vi "Generate Simulated Data.vi"(6 "Acquisition":refnum<queue>, 8 "error in (no error)":errorcluster, 10 "Longueur d'onde":dbl) -> (0 "error out":errorcluster, 2 "Data Out":variant[](array[variant]), 3 "Disconnected":bool=TRUE)   [LabVIEW 2018, in "Acquisition.lvlib"]
doc: "Generates sample waveforms according to the signal type in the HW Config input."
uses:
  Acquisition.lvlib
  support/Message Queue/Message Cluster.ctl
  <vilib>/DAQmx/write.llb/DAQmx Write (Digital 1D Bool NChan 1Samp 1Line).vi
  <vilib>/DAQmx/read.llb/DAQmx Read (Analog 1D Wfm NChan NSamp).vi
  <vilib>/Analysis/baseanly.llb/Mean (DBL).vi
  <vilib>/Analysis/2dsp.llb/2D Convolution (DBL).vi
  <vilib>/DAQmx/create/channels.llb/DAQmx Create Channel (DO-Digital Output).vi
  <vilib>/DAQmx/miscellaneous.llb/DAQmx Fill In Error Info.vi
  <vilib>/DAQmx/create/channels.llb/DAQmx Create Channel (AI-Voltage-Basic).vi
  <vilib>/DAQmx/configure/timing.llb/DAQmx Timing (Sample Clock).vi
  support/Message Queue/Enqueue Message (Single).vi
  GlobalVariable/GlobalPowerByTime.vi
  GlobalVariable/GlobalSet0.vi
  GlobalVariable/GlobalPosYbyTime.vi
  GlobalVariable/GlobalPosXbyTime.vi
  GlobalVariable/GlobalProfileByTime.vi
  GlobalVariable/Globalt0.vi
  GlobalVariable/GlobalTensionByTime.vi
  GlobalVariable/GlobalTemperatureByTime.vi
  GlobalVariable/GlobalTimeStep.vi
  <vilib>/gmath/interp.llb/Create Mesh Grid (2D) (x,y arrays).vi
  <vilib>/Analysis/NI_AALBase.lvlib
  support/Message Queue/Message Queue.lvlib
  <vilib>/gmath/NI_Gmath.lvlib
  <vilib>/Analysis/NI_AALPro.lvlib
  <resource>/objmgr/daqmx.rc
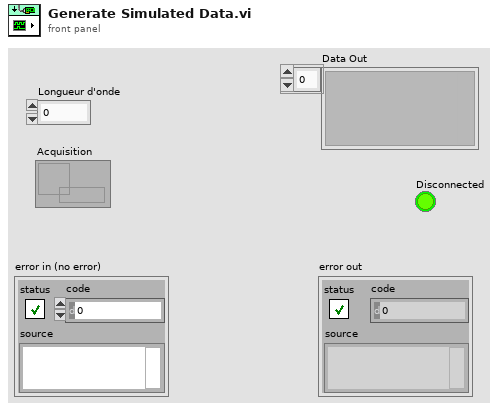
[diagram p1: front panel]
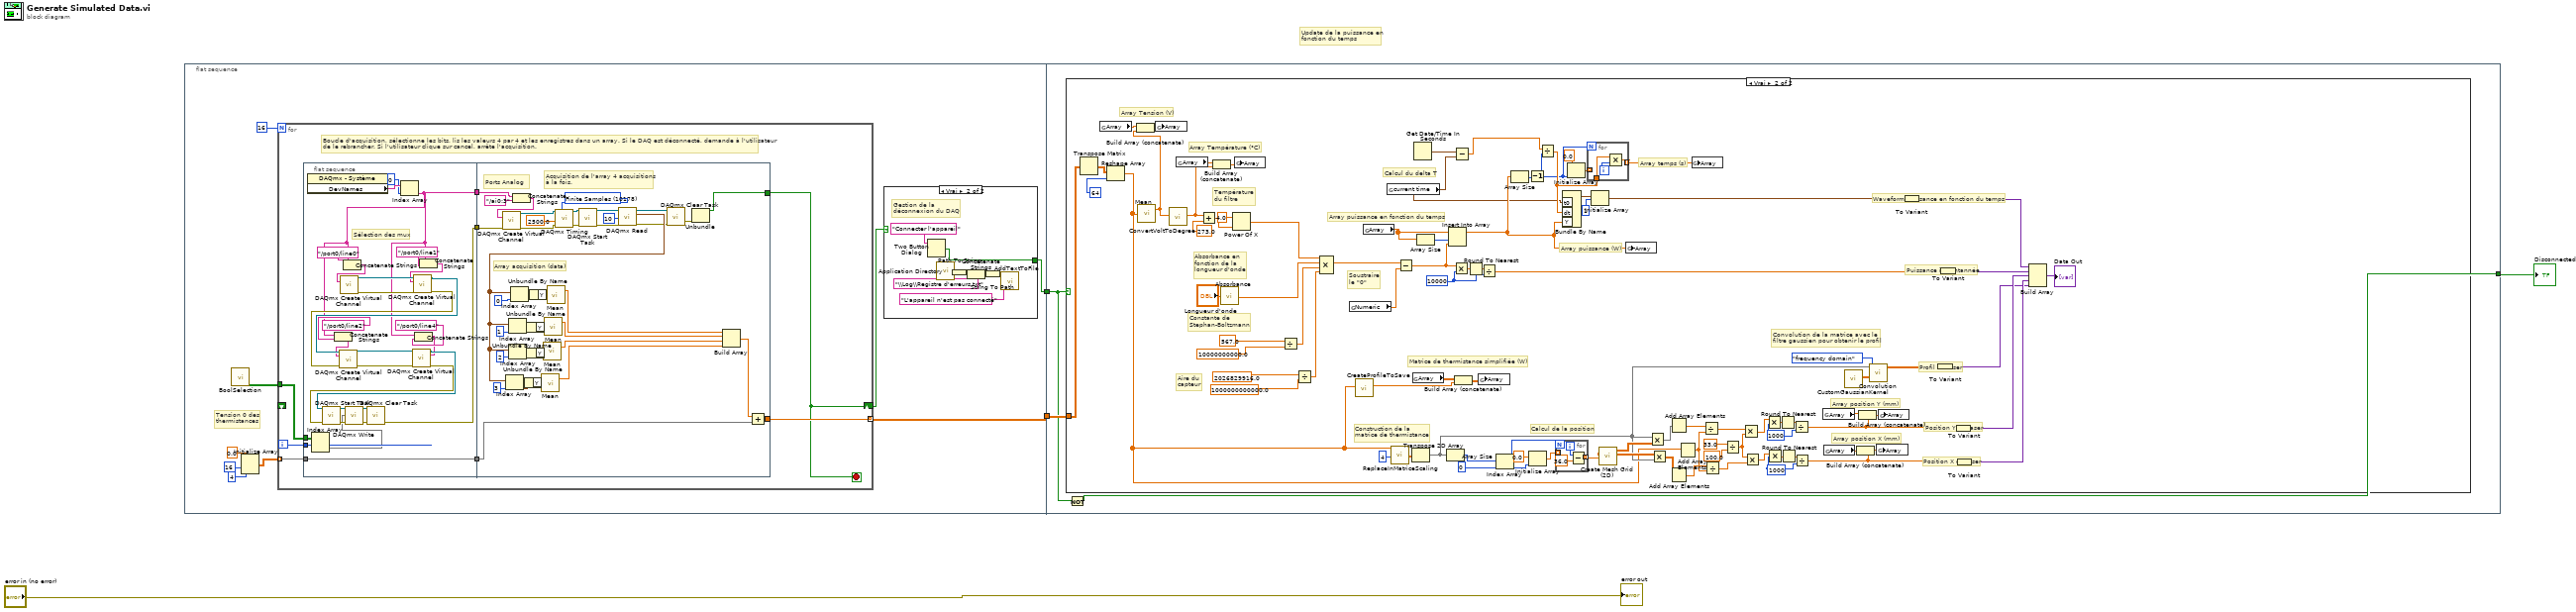
[diagram p0: block diagram]
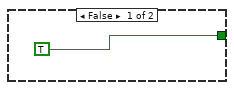
[diagram p2: hidden frame]
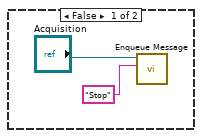
[diagram p3: hidden frame]
diagram:
  # "Update de la puissance en\nfonction du temps"
  n1 = flat-sequence {
    tunnel: [w11] -> w3
    tunnel: [w10] -> w2
    tunnel: w3 -> [w98]
    tunnel: w2 -> [w97]
    tunnel: [w96] -> w1
    frame #0 {
      # "Tension 0 des \nthermistances"
      n2 = call "BoolSelection.vi"() -> ("BoolSelection"=w12:bool[][])  [unwired: 11 in]
      n3 = Initialize Array(0.0 ("element"), 16 ("dimension size"), 4 ("dimension size")) -> (w6:dbl[][])
      n4 = for {
        N: 16 -> [_]
        tunnel: w12 -> [w28]
        tunnel: w6 -> [w26] mode=indexing
        tunnel: [w25] -> w11 mode=indexing
        shift-right: [w24] -> w5
        shift-left: _ -> [_]
        i -> [w29]
        stop <- w24 stop-if-true
        # "Boucle d'acquisition, sélectionne les bits, lis les valeurs 4 par 4 et les enregistres dans un array. Si le DAQ est déconnecté, demande à l'utilisateur \nde le rebrancher. Si l'utilisateur clique sur cancel, arrête l'acquisition."
        n5 = flat-sequence {
          tunnel: w29 -> [w44]
          tunnel: [w55] -> w30
          tunnel: w28 -> [w43]
          tunnel: [w42] -> w27
          tunnel: w26 -> [w42]
          tunnel: [w31] -> w23
          tunnel: w30 -> [w87]
          tunnel: w27 -> [w66]
          tunnel: [w68] -> w25
          tunnel: [w69] -> w24
          tunnel: w23 -> [w63]
          frame #0 {
            # "Sélection des mux"
            n6 = property class="DAQmx - Système"() -> ("DevNames"=w41:tag[])  [unwired: 2 in, 2 out]
            n7 = Index Array(array=w43, index (row)=w44) -> (element=w56:bool[])  [unwired: 1 in]
            n8 = Index Array(array=w41, index=0) -> (element=w31:tag)
            n9 = Concatenate Strings(w31, "/port0/line2" ("string")) -> (w34:string)
            n10 = Concatenate Strings(w31, "/port0/line0" ("string")) -> (w39:string)
            n11 = call-poly <vilib>:"DAQmx Create Virtual Channel.vi"("lines"=w39) -> ("task out"=w51:refnum<k21>, "error out"=w52:errorcluster)  [unwired: 13 in]
            n12 = Concatenate Strings(w31, "/port0/line4" ("string")) -> (w32:string)
            n13 = Concatenate Strings(w31, "/port0/line1" ("string")) -> (w36:string)
            n14 = call-poly <vilib>:"DAQmx Create Virtual Channel.vi"("task in"=w51, "lines"=w36, "error in"=w52) -> ("task out"=w50:refnum<k21>, "error out"=w49:errorcluster)  [unwired: 11 in]
            n15 = call-poly <vilib>:"DAQmx Create Virtual Channel.vi"("task in"=w50, "lines"=w34, "error in"=w49) -> ("task out"=w47:refnum<k21>, "error out"=w48:errorcluster)  [unwired: 11 in]
            n16 = call-poly <vilib>:"DAQmx Create Virtual Channel.vi"("task in"=w47, "lines"=w32, "error in"=w48) -> ("task out"=w46:refnum<k21>, "error out"=w45:errorcluster)  [unwired: 11 in]
            n17 = call <vilib>:"DAQmx Start Task.vi"("task/channels in"=w46, "error in"=w45) -> ("task out"=w57:refnum<k21>, "error out"=w58:errorcluster)  [unwired: 12 in]
            n18 = call-poly <vilib>:"DAQmx Write.vi"("task/channels in"=w57, "data"=w56, "error in"=w58) -> ("task out"=w54:refnum<k21>, "error out"=w53:errorcluster)  [unwired: 10 in, 1 out]
            n19 = call <vilib>:"DAQmx Clear Task.vi"("task in"=w54, "error in"=w53) -> ("error out"=w55:errorcluster)  [unwired: 13 in]
          }
          frame #1 {
            w89 = 10178 items=["Finite Samples"=10178, "Continuous Samples"=10123, "Hardware Timed Single Point"=12522] ("sample mode")
            # "Ports Analog"
            # "Array acquisition (data)"
            # "Acquisition de l'array 4 acquisitions\nà la fois."
            n20 = Concatenate Strings(w63, "/ai0:3" ("string")) -> (w64:string)
            n21 = call-poly <vilib>:"DAQmx Create Virtual Channel.vi"("physical channels"=w64, "error in"=w87) -> ("task out"=w94:refnum<k21>, "error out"=w93:errorcluster)  [unwired: 12 in]
            n22 = call-poly <vilib>:"DAQmx Timing.vi"("task/channels in"=w94, "sample mode"=w89, "rate"=2500.0, "error in"=w93) -> ("task out"=w90:refnum<k21>, "error out"=w91:errorcluster)  [unwired: 10 in]
            n23 = call <vilib>:"DAQmx Start Task.vi"("task/channels in"=w90, "error in"=w91) -> ("task out"=w92:refnum<k21>, "error out"=w95:errorcluster)  [unwired: 12 in]
            n24 = call-poly <vilib>:"DAQmx Read.vi"("task/channels in"=w92, "number of samples per channel"=10, "error in"=w95) -> ("task out"=w71:refnum<k21>, "data"=w80:waveform(dbl)[], "error out"=w70:errorcluster)  [unwired: 10 in]
            n25 = Index Array(array=w80, index=3) -> (element=w76:waveform(dbl))
            n26 = Index Array(array=w80, index=1) -> (element=w78:waveform(dbl))
            n27 = Index Array(array=w80, index=2) -> (element=w77:waveform(dbl))
            n28 = Index Array(array=w80, index=0) -> (element=w79:waveform(dbl))
            n29 = Unbundle By Name(w76) -> ("Y"=w72:dbl[])
            n30 = Unbundle By Name(w78) -> ("Y"=w74:dbl[])
            n31 = Unbundle By Name(w77) -> ("Y"=w73:dbl[])
            n32 = Unbundle By Name(w79) -> ("Y"=w75:dbl[])
            n33 = call-poly <vilib>:"Mean.vi"("X"=w72) -> ("mean"=w59:dbl)  [unwired: 1 out]
            n34 = call-poly <vilib>:"Mean.vi"("X"=w73) -> ("mean"=w60:dbl)  [unwired: 1 out]
            n35 = call-poly <vilib>:"Mean.vi"("X"=w74) -> ("mean"=w61:dbl)  [unwired: 1 out]
            n36 = call-poly <vilib>:"Mean.vi"("X"=w75) -> ("mean"=w62:dbl)  [unwired: 1 out]
            n37 = call <vilib>:"DAQmx Clear Task.vi"("task in"=w71, "error in"=w70) -> ("error out"=w85:errorcluster)  [unwired: 13 in]
            n38 = Unbundle(w85) -> ("status"=w69:bool)  [unwired: 2 out]
            n39 = Build Array(w62, w61, w60, w59) -> (w67:dbl[])
            n40 = Add(x=w67, y=w66) -> (x+y=w68:dbl[])
          }
        }
      }
      n41 = case shown="Vrai" w5 {
        tunnel: [TRUE w22] -> w10
        frame False {
        }
        frame True {
          # "Gestion de la \ndéconnexion du DAQ"
          n42 = Two Button Dialog(message="Connecter l'appareil") -> (T button?=w22:bool)  [unwired: 2 in]
          n43 = call <vilib>:"Application Directory.vi"() -> ("Application Directory"=w19:path)
          n44 = Path To String(path=w19) -> (string=w20:string)
          n45 = Concatenate Strings(w20, "\\Log\\Registre d'erreurs.txt") -> (w21:string)
          n46 = String To Path(string=w21) -> (path=w17:path)
          n47 = call "AddTextToFile.vi"("Ajouter du texte"="L'appareil n'est pas connecté", "Fichier"=w17) -> ()  [unwired: 10 in]
        }
      }
    }
    frame #1 {
      n48 = case shown="Vrai" w97 {
        tunnel: w98 -> [_ w128]
        frame False {
          n49 = call-poly "Enqueue Message.vi"("Message"="Stop", "Message Queue"="Acquisition") -> ()  [unwired: 8 in, 2 out]
        }
        frame True {
          w140 = 1000
          w144 = 1000
          w150 = 10000
          # "Array position X (mm)"
          # "Array position Y (mm)"
          # "Array Température (°C)"
          # "Array Tension (V)"
          # "Calcul du delta T"
          # "Matrice de thermistance simplifiée (W)"
          # "Soustraire\nle \"0\""
          # "Constante de \nStephan-Boltzmann"
          # "Absorbance en\nfonction de la \nlongueur d'onde"
          # "Température \ndu filtre"
          # "Aire du\ncapteur"
          # "Calcul de la position"
          # "Construction de la \nmatrice de thermistance"
          # "Position X du laser"
          # "Position Y du laser"
          # "Profil du laser"
          # "Puissance instantannée"
          # "Waveform puissance en fonction du temps"
          # "Array puissance (W)"
          # "Array temps (s)"
          # "Convolution de la matrice avec le \nfiltre gaussien pour obtenir le profil"
          # "Array puissance en fonction du temps"
          n50 = Transpose Matrix(1:w128) -> (0:w129:dbl[][])
          n51 = global read "GlobalTensionByTime.vi" "Array"() -> (w106:dbl[])
          n52 = Reshape Array(w129, 64 ("dimension size")) -> (w123:dbl[])
          n53 = call-poly <vilib>:"Mean.vi"("X"=w123) -> ("mean"=w104:dbl)  [unwired: 1 out]
          n54 = Build Array (concatenate)(w106, w104) -> (w105:dbl[])
          n55 = global write "GlobalTensionByTime.vi" "Array"(w105) -> ()
          n56 = call "ConvertVoltToDegree.vi"("Tension"=w104) -> ("Température"=w101:dbl)  [unwired: 10 in]
          n57 = global read "GlobalTemperatureByTime.vi" "Array"() -> (w102:dbl[])
          n58 = Add(x=w101, y=273.0) -> (x+y=w179:dbl)
          n59 = Build Array (concatenate)(w102, w101) -> (w103:dbl[])
          n60 = call "Absorbance.vi"("Longueur d'onde"="Longueur d'onde") -> ("absorbance"=w132:dbl)  [unwired: 10 in]
          n61 = Power Of X(1:w179, 2:4.0 ("y")) -> (0:w131:dbl)
          n62 = global write "GlobalTemperatureByTime.vi" "Array"(w103) -> ()
          n63 = Divide(x=567.0, y=10000000000.0) -> (x/y=w133:dbl)
          n64 = Divide(x=2026829916.0, y=1000000000000.0) -> (x/y=w134:dbl)
          n65 = Compound Arithmetic op=MULTIPLY(w131, w132, w133, w134) -> (w127:dbl)
          n66 = global read "GlobalSet0.vi" "Numeric"() -> (w126:dbl)
          n67 = call "CreateProfileToSave.vi"("Input Array"=w123) -> ("Ouput array"=w113:dbl[])  [unwired: 10 in]
          n68 = global read "GlobalPowerByTime.vi" "Array"() -> (w191:dbl[])
          n69 = global read "Globalt0.vi" "current time"() -> (w108:timestamp)
          n70 = call "ReplaceInMatriceScaling.vi"("Input Scaling"=4, "Input Array"=w123) -> ("Output Array"=w186:dbl[][])  [unwired: 9 in]
          n71 = Subtract(x=w127, y=w126) -> (x-y=w125:dbl)
          n72 = Transpose 2D Array(2D array=w186) -> (transposed array=w124:dbl[][])
          n73 = global read "GlobalProfileByTime.vi" "Array"() -> (w112:dbl[][])
          n74 = Get Date/Time In Seconds() -> (seconds since 1Jan1904=w109:timestamp)
          n75 = Array Size(array=w191) -> (size(s)=w190:i32)
          n76 = Array Size(array=w124) -> (size(s)=w173:i32[])
          n77 = Insert Into Array(array=w191, index=w190, new element=w125) -> (w122:dbl[])
          n78 = Multiply(x=w125, y=w150) -> (x*y=w151:dbl)
          n79 = Subtract(x=w109, y=w108) -> (x-y=w107:dbl)
          n80 = Build Array (concatenate)(w112, w113) -> (w114:dbl[][])
          n81 = Round To Nearest(number=w151) -> (nearest integer value=w149:dbl)
          n82 = global write "GlobalProfileByTime.vi" "Array"(w114) -> ()
          n83 = Divide(x=w149, y=w150) -> (x/y=w145:dbl)
          n84 = Index Array(array=w173, index=0) -> (element=w168:i32)
          n85 = Array Size(array=w122) -> (size(s)=w111:i32)
          n86 = Decrement(x=w111) -> (x-1=w110:i32)
          n87 = Initialize Array(0.0 ("element"), w168) -> (w170:dbl[])
          n88 = Divide(x=w107, y=w110) -> (x/y=w184:dbl)
          n89 = for {
            N: w168 -> [_]
            tunnel: w170 -> [_] mode=indexing
            tunnel: [w192] -> w165 mode=indexing
            i -> [w193]
            n90 = Subtract(x=w193, y=36.0) -> (x-y=w192:dbl)
          }
          n91 = Bundle By Name("t0"=w108, "dt"=w184, "Y"=w122) -> (w188:waveform(dbl))  [unwired: 1 in]
          n92 = Initialize Array(0.0 ("element"), w110) -> (w182:dbl[])
          n93 = for {
            N: w110 -> [_]
            tunnel: w184 -> [w196]
            tunnel: w182 -> [_] mode=indexing
            tunnel: [w195] -> w121 mode=indexing
            i -> [w197]
            n94 = Multiply(x=w196, y=w197) -> (x*y=w195:dbl)
          }
          n95 = Initialize Array(w188, 1) -> (w154:waveform(dbl)[])
          n96 = call-poly <vilib>:"Create Mesh Grid (2D).vi"("y domain"=w165, "x domain"=w165) -> ("Y"=w164:dbl[][], "X"=w169:dbl[][])  [unwired: 7 in, 1 out]
          n97 = global write "GlobalPowerByTime.vi" "Array"(w122) -> ()
          n98 = Multiply(x=w124, y=w169) -> (x*y=w167:dbl[][])
          n99 = Multiply(x=w164, y=w124) -> (x*y=w163:dbl[][])
          n100 = Add Array Elements(numeric array=w167) -> (sum=w166:dbl)
          n101 = Add Array Elements(numeric array=w163) -> (sum=w162:dbl)
          n102 = Add Array Elements(numeric array=w123) -> (sum=w161:dbl)
          n103 = global write "GlobalTimeStep.vi" "Array"(w121) -> ()
          n104 = Divide(x=w166, y=w161) -> (x/y=w159:dbl)
          n105 = Divide(x=w162, y=w161) -> (x/y=w160:dbl)
          n106 = Divide(x=33.0, y=100.0) -> (x/y=w158:dbl)
          n107 = Multiply(x=w159, y=w158) -> (x*y=w141:dbl)
          n108 = Multiply(x=w158, y=w160) -> (x*y=w137:dbl)
          n109 = Multiply(x=w141, y=w144) -> (x*y=w143:dbl)
          n110 = Multiply(x=w137, y=w140) -> (x*y=w139:dbl)
          n111 = Round To Nearest(number=w143) -> (nearest integer value=w142:dbl)
          n112 = Round To Nearest(number=w139) -> (nearest integer value=w138:dbl)
          n113 = Divide(x=w142, y=w144) -> (x/y=w115:dbl)
          n114 = Divide(x=w138, y=w140) -> (x/y=w119:dbl)
          n115 = global read "GlobalPosXbyTime.vi" "Array"() -> (w116:dbl[])
          n116 = global read "GlobalPosYbyTime.vi" "Array"() -> (w120:dbl[])
          n117 = call "CustomGaussianKernel.vi"() -> ("array"=w181:dbl[][])  [unwired: 11 in]
          n118 = Build Array (concatenate)(w120, w119) -> (w118:dbl[])
          n119 = Build Array (concatenate)(w116, w115) -> (w117:dbl[])
          n120 = call-poly <vilib>:"Convolution.vi"("algorithm"=enum32{"direct", "frequency domain"}."frequency domain", "Y"=w181, "X"=w124) -> ("X * Y"=w135:dbl[][])  [unwired: 7 in, 1 out]
          n121 = global write "GlobalPosYbyTime.vi" "Array"(w118) -> ()
          n122 = global write "GlobalPosXbyTime.vi" "Array"(w117) -> ()
          n123 = To Variant(anything=w154) -> (Variant=w153:variant)
          n124 = To Variant(anything=w135) -> (Variant=w136:variant)
          n125 = To Variant(anything=w145) -> (Variant=w146:variant)
          n126 = To Variant(anything=w115) -> (Variant=w147:variant)
          n127 = To Variant(anything=w119) -> (Variant=w148:variant)
          n128 = Build Array(w153, w146, w147, w148, w136) -> (→"Data Out":variant[])
        }
      }
      n129 = Not(x=w97) -> (.not. x?=w96:bool)
    }
  }
  "error out" <- "error in (no error)"
  "Disconnected" <- w1
